vi "串口配置.vi"() -> ()   [LabVIEW 2016, in "质控单元V4.lvlib"]
panel:
  in  "Tab Control 2":enum32{"Comm Settings"}(tab)
  in  "关闭":bool
  in  "Open":bool
  in  "Close":bool
  in  "Type":enum16{"Serial", "TCP"}(ring) caption="Connection Type"
  out "Tab Control":enum32{"Page 1", "Page 2"}(tab)
  in  "Retries":i32=1
  in  "Timeout (ms)":u32=1000
  in  "Flow Control":u16(ring) items=["None", "XON/XOFF", "RTS/CTS", "XON/XOFF & RTS/CTS", "DTR/DSR", "XON/XOFF & DTR/DSR"]
  in  "Parity":u16(ring) items=["None", "Odd", "Even", "Mark", "Space"]
  in  "Stop Bits":u16(ring)=10 items=["1.0"=10, "1.5"=15, "2.0"=20]
  in  "Baud Rate (bps)":u32(ring)=115200 items=["9600"=9600, "19200"=19200, "38400"=38400, "57600"=57600, "115200"=115200, "460800"=460800, "921600"=921600]
  in  "Slave Address":u8=1
  in  "Mode":enum16{"RTU", "ASCII"}(ring)
  in  "COM Port":refnum<visa-resource-name>="COM8"
  in  "TCP_Port":u16=502 caption="Port"
  in  "IP Address":string="192.168.1.207"
  in  "TCP_Timeout":i32=1000 caption="Timeout (ms)"
  in  "TCP_Slave ID":u8=255 caption="Slave ID" format="%.0x"
  # "Communication Settngs"
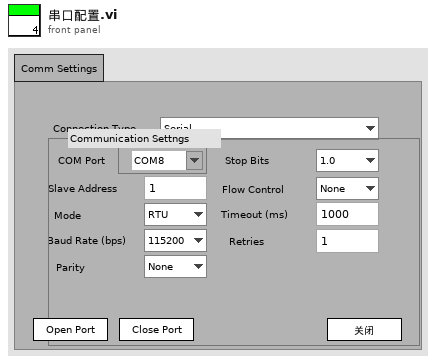
[diagram p1: front panel]
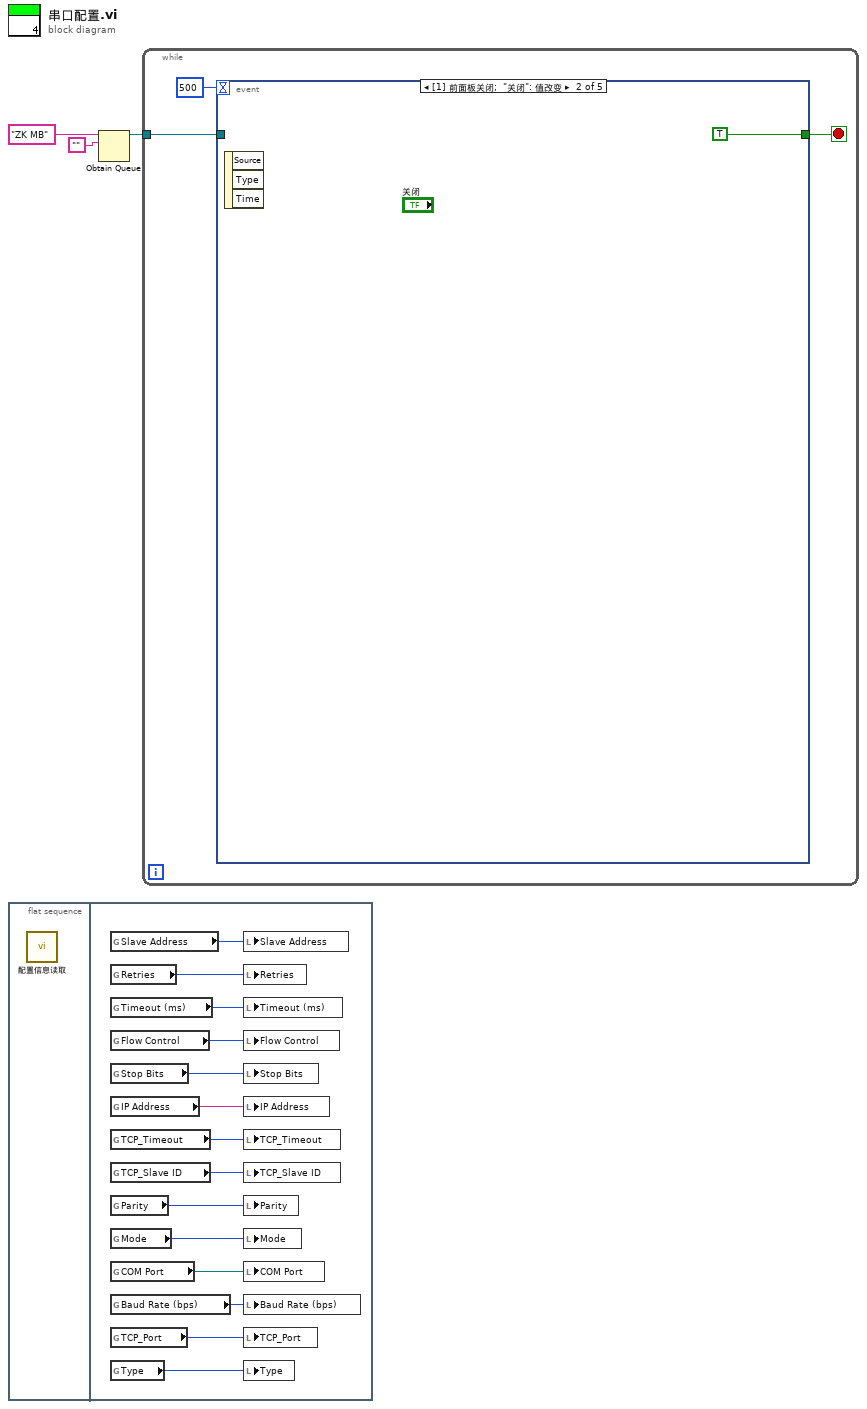
[diagram p0: block diagram]
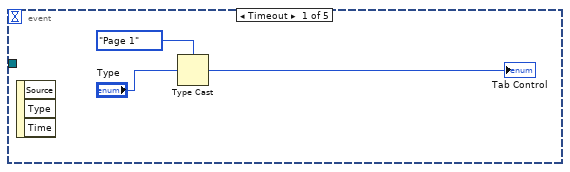
[diagram p2: hidden frame]
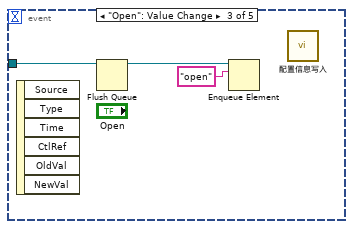
[diagram p3: hidden frame]
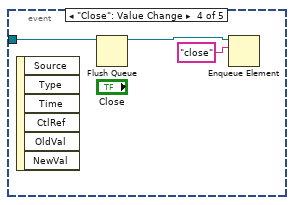
[diagram p4: hidden frame]
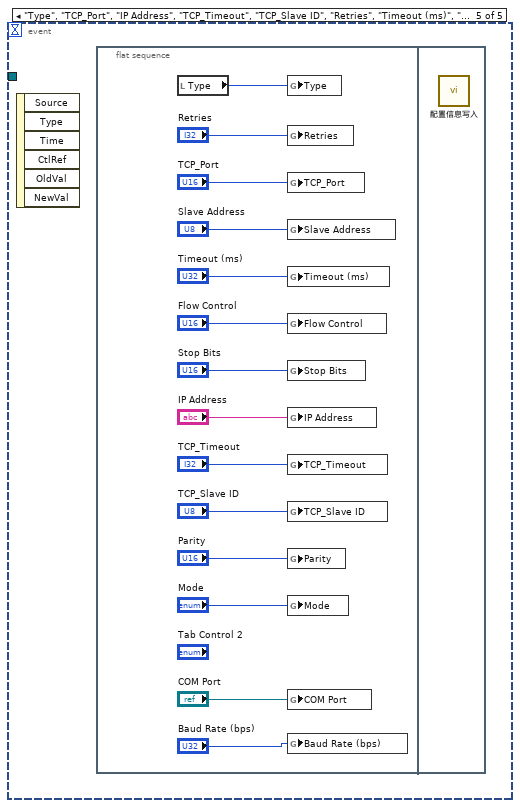
[diagram p5: hidden frame]
diagram:
  n1 = flat-sequence {
    frame #0 {
      n2 = call "配置信息读取.vi"() -> ()  [unwired: 11 in, 1 out]
    }
    frame #1 {
      n3 = global read "ZK断电保存全局变量.vi" "Slave Address"() -> (w5:u8)
      n4 = global read "ZK断电保存全局变量.vi" "Retries"() -> (w6:i32)
      n5 = global read "ZK断电保存全局变量.vi" "Timeout (ms)"() -> (w7:u32)
      n6 = global read "ZK断电保存全局变量.vi" "Flow Control"() -> (w8:u16)
      n7 = global read "ZK断电保存全局变量.vi" "Stop Bits"() -> (w9:u16)
      n8 = global read "ZK断电保存全局变量.vi" "IP Address"() -> (w10:string)
      n9 = global read "ZK断电保存全局变量.vi" "TCP_Timeout"() -> (w11:i32)
      n10 = global read "ZK断电保存全局变量.vi" "TCP_Slave ID"() -> (w12:u8)
      n11 = global read "ZK断电保存全局变量.vi" "Parity"() -> (w13:u16)
      n12 = global read "ZK断电保存全局变量.vi" "Mode"() -> (w14:enum16{"RTU", "ASCII"})
      n13 = global read "ZK断电保存全局变量.vi" "COM Port"() -> (w15:refnum<visa-resource-name>)
      n14 = global read "ZK断电保存全局变量.vi" "Baud Rate (bps)"() -> (w16:u32)
      n15 = global read "ZK断电保存全局变量.vi" "TCP_Port"() -> (w4:u16)
      n16 = global read "ZK断电保存全局变量.vi" "Type"() -> (w17:enum16{"Serial", "TCP"})
      n17 = local write "Slave Address"(w5) -> ()
      n18 = local write "Retries"(w6) -> ()
      n19 = local write "Timeout (ms)"(w7) -> ()
      n20 = local write "Flow Control"(w8) -> ()
      n21 = local write "Stop Bits"(w9) -> ()
      n22 = local write "IP Address"(w10) -> ()
      n23 = local write "TCP_Timeout"(w11) -> ()
      n24 = local write "TCP_Slave ID"(w12) -> ()
      n25 = local write "Parity"(w13) -> ()
      n26 = local write "Mode"(w14) -> ()
      n27 = local write "COM Port"(w15) -> ()
      n28 = local write "Baud Rate (bps)"(w16) -> ()
      n29 = local write "TCP_Port"(w4) -> ()
      n30 = local write "Type"(w17) -> ()
    }
  }
  n31 = Obtain Queue(name (unnamed)="ZK MB" ("名称（未命名）"), element data type="") -> (queue out=w1:refnum<queue>)  [unwired: 3 in, 2 out]
  n32 = while {
    tunnel: w1 -> [w18]
    stop <- w20 stop-if-true
    n33 = event shown="[1] 前面板关闭;  \"关闭\": 值改变" {
      selector: _ -> [_ _ _ _ _]
      dyn-events: _ -> [_ _ _ _ _]
      timeout: 500 -> [_ _ _ _ _]
      tunnel: [_ TRUE _ _ _] -> w20
      tunnel: w18 -> [_ _ w27 w28 _]
      event Timeout {
        n34 = event-data() -> ()  [unwired: 1 in, 3 out]
        n35 = Type Cast(type=enum32{"Page 1", "Page 2"}."Page 1" ("Tab Control"), x="Type") -> (*(type *) &x=→"Tab Control":enum32{"Page 1", "Page 2"})
      }
      event Panel Close; "关闭": Value Change {
        n36 = event-data() -> ()  [unwired: 1 in, 3 out]
      }
      event "Open": Value Change {
        n37 = event-data() -> ()  [unwired: 1 in, 6 out]
        n38 = Flush Queue(queue=w27) -> (queue out=w26:refnum<queue>)  [unwired: 1 in, 2 out]
        n39 = Enqueue Element(queue=w26, element="open" ("元素")) -> ()  [unwired: 2 in, 3 out]
        n40 = call "配置信息写入.vi"() -> ()  [unwired: 11 in, 1 out]
      }
      event "Close": Value Change {
        n41 = event-data() -> ()  [unwired: 1 in, 6 out]
        n42 = Flush Queue(queue=w28) -> (queue out=w30:refnum<queue>)  [unwired: 1 in, 2 out]
        n43 = Enqueue Element(queue=w30, element="close" ("元素")) -> ()  [unwired: 2 in, 3 out]
      }
      event "Type", "TCP_Port", "IP Address", "TCP_Timeout", "TCP_Slave ID", "Retries", "Timeout (ms)", "Flow Control", "Parity", "Stop Bits", "Baud Rate (bps)", "Slave Address", "Mode", "COM Port": Value Change {
        n44 = event-data() -> ()  [unwired: 1 in, 6 out]
        n45 = flat-sequence {
          frame #0 {
            n46 = local read "Type"() -> (w32:enum16{"Serial", "TCP"})
            n47 = global write "ZK断电保存全局变量.vi" "Type"(w32) -> ()
            n48 = global write "ZK断电保存全局变量.vi" "Retries"("Retries") -> ()
            n49 = global write "ZK断电保存全局变量.vi" "TCP_Port"("TCP_Port") -> ()
            n50 = global write "ZK断电保存全局变量.vi" "Slave Address"("Slave Address") -> ()
            n51 = global write "ZK断电保存全局变量.vi" "Timeout (ms)"("Timeout (ms)") -> ()
            n52 = global write "ZK断电保存全局变量.vi" "Flow Control"("Flow Control") -> ()
            n53 = global write "ZK断电保存全局变量.vi" "Stop Bits"("Stop Bits") -> ()
            n54 = global write "ZK断电保存全局变量.vi" "IP Address"("IP Address") -> ()
            n55 = global write "ZK断电保存全局变量.vi" "TCP_Timeout"("TCP_Timeout") -> ()
            n56 = global write "ZK断电保存全局变量.vi" "TCP_Slave ID"("TCP_Slave ID") -> ()
            n57 = global write "ZK断电保存全局变量.vi" "Parity"("Parity") -> ()
            n58 = global write "ZK断电保存全局变量.vi" "Mode"("Mode") -> ()
            n59 = global write "ZK断电保存全局变量.vi" "COM Port"("COM Port") -> ()
            n60 = global write "ZK断电保存全局变量.vi" "Baud Rate (bps)"("Baud Rate (bps)") -> ()
          }
          frame #1 {
            n61 = call "配置信息写入.vi"() -> ()  [unwired: 11 in, 1 out]
          }
        }
      }
    }
  }
